vi "Active Output Results.vi"(7 "step name (\"\")":string, 8 "error in":errorcluster, 9 "Result":dbl=nan format="%.3g", 10 "test case":T2(ring), 11 "Sequence Context":refnum<k7>) -> (0 "error out":errorcluster, 3 "Sequence Context dup":refnum<k7>)   [LabVIEW 2010]
doc: "This function transfers a single Compare Data Test (CDT) record to the current TestStand sequence step."
uses:
  Generic/TestConsole/Test Criteria Control.ctl
panel:
  in  "Acceptance Criteria":T1
  in  "Test Criteria":T1=[["", "Load 1 Resistance", "", "9900.0", "10100.0", "ohms", "GELE", "%.1f", "%.1f", "Load1"], ["", "Load 1 DC Offset", "", "-15.0", "15.0", "mV", "GELE", "%.1f", "%.1f", "Offset1"], ["", "Load 3 Resistance", "", "494.0", "504.0", "ohms", "GELE", "%.1f", "%.1f", "Load3"], ["", "Load 3 DC Offset", "", "-15.0", "15.0", "mV", "GELE", "%.1f", "%.1f", "Offset3"], ["", "Load 25 Resistance", "", "247.0", "252.0", "ohms", "GELE", "%.1f", "%.1f", "Load25"], ["", "Load 25 DC Offset", "", "-15.0", "15.0", "mV", "GELE", "%.1f", "%.1f", "Offset25"], ["", "Tegam1 Trimmed Offset Error 10 V", "", "-100.0", "100.0", "uV", "GELE", "%.1f", "%.1f", "T1_10V"], ["", "Tegam2 Trimmed Offset Error 10 V", "", "-100.0", "100.0", "uV", "GELE", "%.1f", "%.1f", "T2_10V"], ["", "Tegam1 Trimmed Offset Error 100 V", "", "-100.0", "100.0", "uV", "GELE", "%.1f", "%.1f", "T1_100V"], ["", "Tegam2 Trimmed Offset Error 100 V", "", "-100.0", "100.0", "uV", "GELE", "%.1f", "%.1f", "T2_100V"], ["", "VBAT Level", "", "3.75", "4.20", "V", "GELE", "%.2f", "%.2f", "VBAT"], ["", "Far Field Comms at (22, 0, 0)", "", "90", "100", "%", "GELE", "%.0f", "%.0f", "FF Comm"], ["", "Near Field Comms at (0, 0, 0)", "", "80", "100", "%", "GELE", "%.0f", "%.0f", "NF Comm"], ["", "Comm Failures at (0, 0, 0) after Magnet Shutdown", "", "100", "", "%", "EQ", "%.0f", "%.0f", "Comm Fail"]]
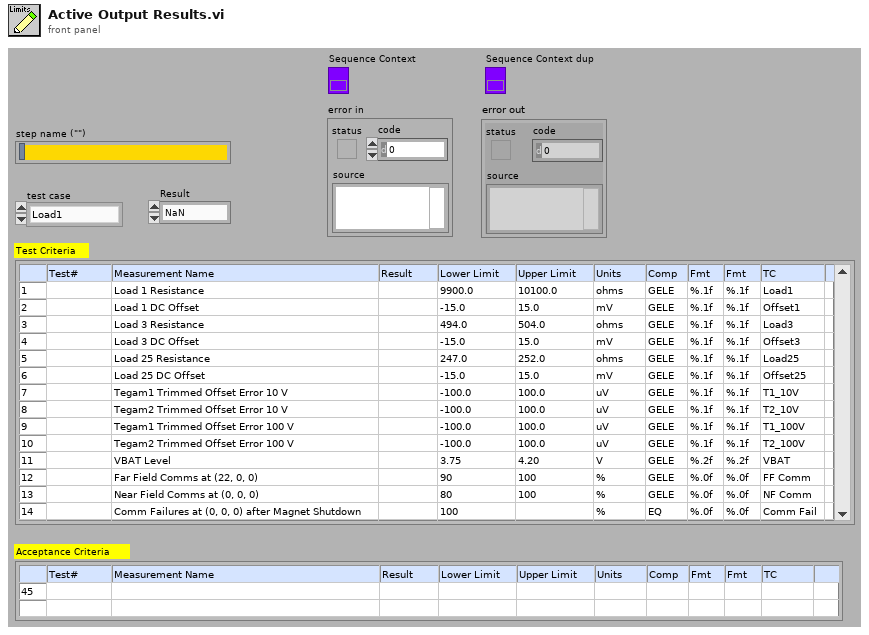
[diagram p1: front panel]
types:
  T1 = typedef "Test Criteria Control.ctl" = string[][]
  T2 = enum16{"Load1", "Offset1", "Load3", "Offset3", "Load25", "Offset25", "T1_10V", "T2_10V", "T1_100V", "T2_100V", "FF Comm", "NF Comm", "Comm Fail", "VBAT"}
  T3 = typedef "TestStand_Result Control.ctl" = cluster{"Measurement Name":string, "Result":dbl, "Low Limit":dbl, "High Limit":dbl, "Units":string, "Comp":string, "DataFmt":string, "LimitFmt":string}
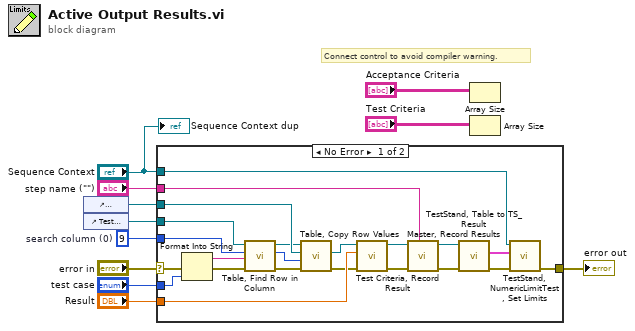
[diagram p0: block diagram]
diagram:
  w2 = 9  # search column (0)
  # "Connect control to avoid compiler warning."
  n1 = control-ref of="Acceptance Criteria"() -> (w3:refnum<vi>)
  n2 = control-ref of="Test Criteria"() -> (w6:refnum<vi>)
  n3 = case shown="No Error" "error in" {
    selector: "error in" -> [w31 w34]
    tunnel: [w30 w34] -> w11
    tunnel: "Sequence Context" -> [w27 _]
    tunnel: "test case" -> [w29 _]
    tunnel: w6 -> [w28 _]
    tunnel: "Result" -> [w21 _]
    tunnel: w3 -> [w20 _]
    tunnel: w2 -> [w16 _]
    tunnel: "step name (\"\")" -> [w13 _]
    frame No Error {
      n4 = Format Into String(error in=w31, w29) -> (resulting string=w33:string, error out=w32:errorcluster)  [unwired: 2 in]
      n5 = call "Table, Find Row in Column.vi"("error in"=w32, "search key"=w33, "search column (0)"=w16, "Tbl Refnum"=w28) -> ("error out"=w19:errorcluster, "row index"=w12:i32, "Tbl Refnum out"=w17:refnum<vi>)  [unwired: 4 in, 1 out]
      n6 = call "Table, Copy Row Values.vi"("error in"=w19, "row (0)"=w12, "Tbl Refnum Dst"=w20, "Tbl Refnum Src"=w17) -> ("error out"=w18:errorcluster, "Tbl Refnum Dst out"=w14:refnum<vi>)  [unwired: 3 in, 1 out]
      n7 = call "Test Criteria, Record Result.vi"("error in"=w18, "Result"=w21, "Tbl Refnum"=w14) -> ("error out"=w22:errorcluster, "Tbl Refnum out"=w15:refnum<vi>)  [unwired: 6 in, 1 out]
      n8 = call "Master, Record Results.vi"("step name"=w13, "error in"=w22, "Tbl Refnum"=w15) -> ("error out"=w24:errorcluster, "Tbl Refnum dup"=w23:refnum<vi>)  [unwired: 7 in]
      n9 = call "TestStand, Table to TS_Result.vi"("error in"=w24, "Tbl Refnum"=w23) -> ("error out"=w25:errorcluster, "TestStand Result"=w26:T3)  [unwired: 7 in, 1 out]
      n10 = call "TestStand, NumericLimitTest, Set Limits.vi"("error in"=w25, "CDT_type"=w26, "Sequence Context"=w27) -> ("error out"=w30:errorcluster)  [unwired: 7 in, 1 out]
    }
    frame Error {
    }
  }
  "error out" <- w11
  n11 = Array Size(array="Acceptance Criteria") -> ()  [unwired: 1 out]
  n12 = Array Size(array="Test Criteria") -> ()  [unwired: 1 out]
  "Sequence Context dup" <- "Sequence Context"
